vi "Has Arrays.vi"(8 "Error In":errorcluster, 11 "ByteBuffer In":refnum<class "ByteBuffer.lvclass">) -> (0 "Error Out":errorcluster, 2 "Has Arrays":bool, 3 "ByteBuffer Out":refnum<class "ByteBuffer.lvclass">)   [LabVIEW 2015, in "ByteBuffer.lvclass"]
doc: "Tells whether or not this buffer is backed by an accessible byte array."
uses:
  ByteBuffer.lvclass
  ByteBuffer.lvclass/ByteBuffer.ctl
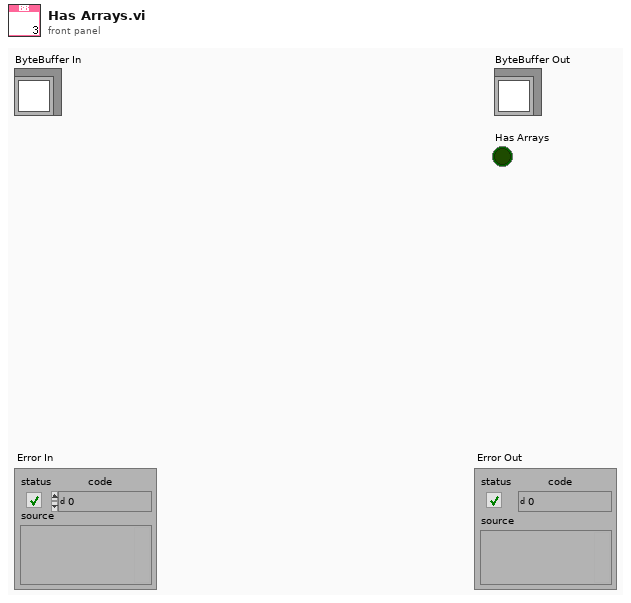
[diagram p1: front panel]
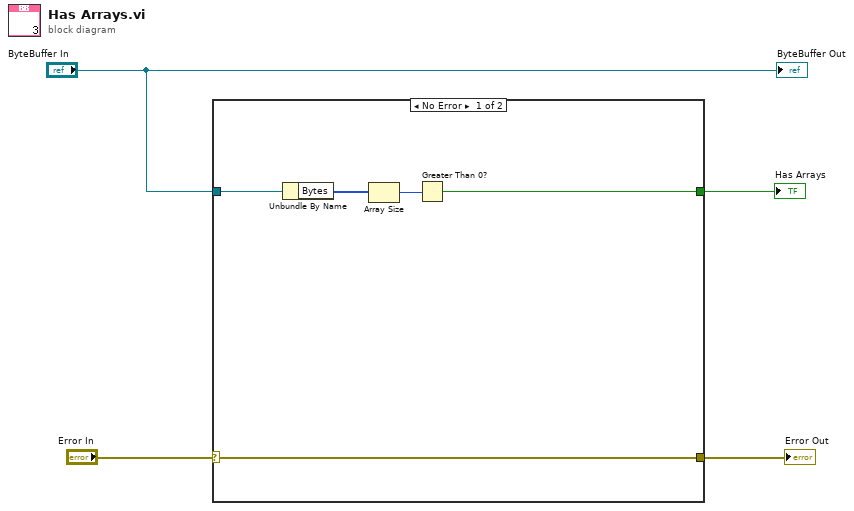
[diagram p0: block diagram]
diagram:
  n1 = case shown="No Error" "Error In" {
    selector: "Error In" -> [w9 w10]
    tunnel: [w9 w10] -> w3
    tunnel: "ByteBuffer In" -> [w8 _]
    tunnel: [w5 _] -> w1
    frame No Error {
      n2 = Unbundle By Name(w8) -> ("Bytes"=w7:u8[])
      n3 = Array Size(array=w7) -> (size(s)=w6:i32)
      n4 = Greater Than 0?(x=w6) -> (x > 0?=w5:bool)
    }
    frame Error {
    }
  }
  "Error Out" <- w3
  "Has Arrays" <- w1
  "ByteBuffer Out" <- "ByteBuffer In"
